vi "format_coords_str.vi"(2 "DEC str":string, 3 "RA str":string) -> (0 "%s DEC":string, 1 "%s RA":string)   [LabVIEW 2010]
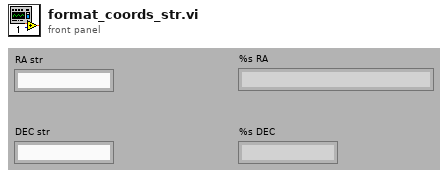
[diagram p1: front panel]
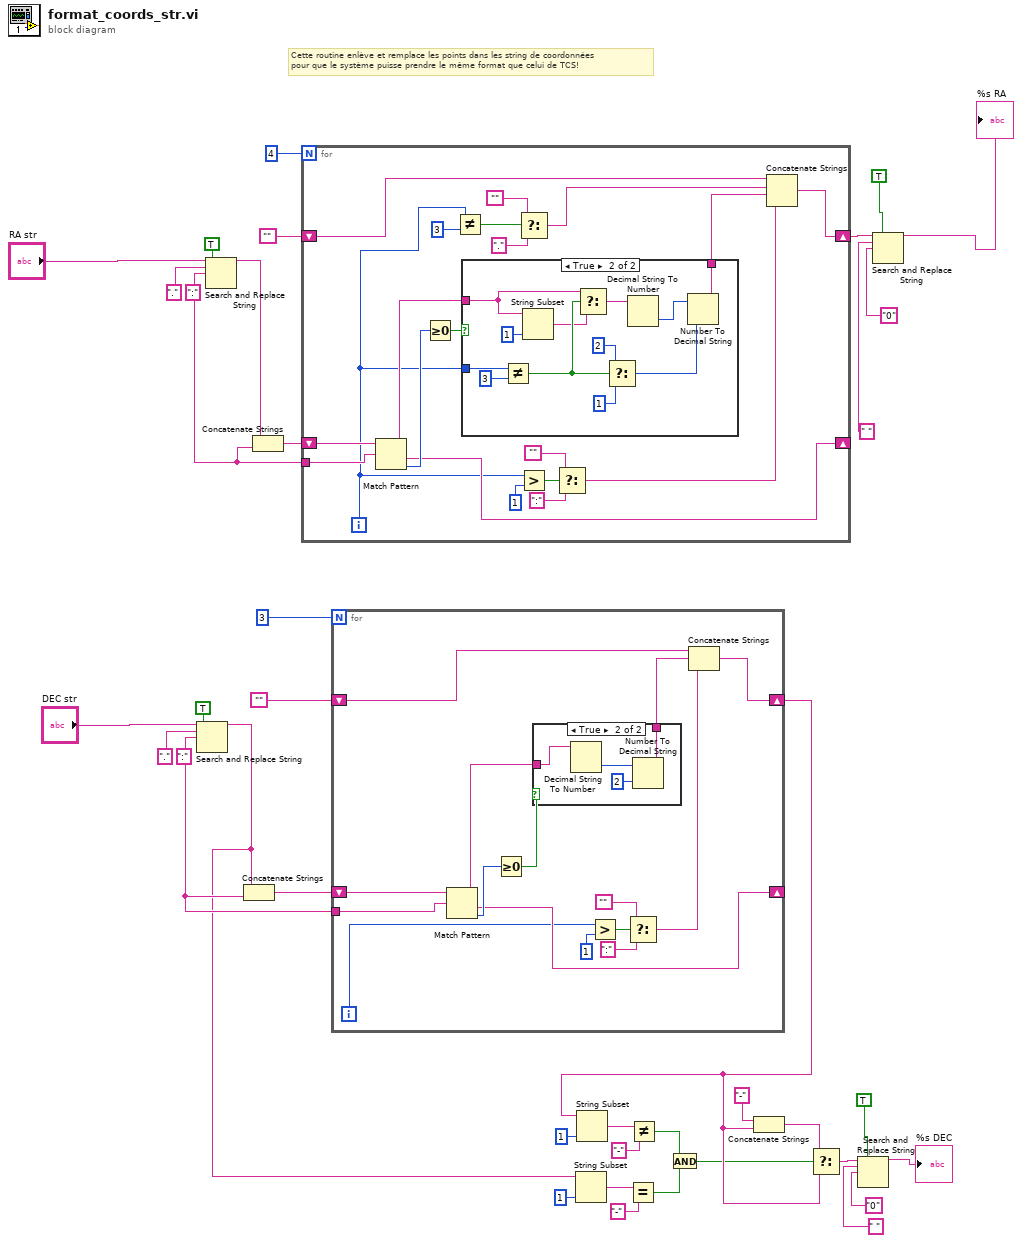
[diagram p0: block diagram]
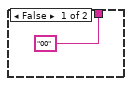
[diagram p2: hidden frame]
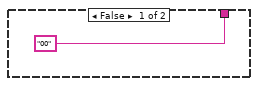
[diagram p3: hidden frame]
diagram:
  w15 = ":" ("replace string (\"\")")
  w31 = ":" ("replace string (\"\")")
  # "Cette routine enlève et remplace les points dans les string de coordonnées \npour que le système puisse prendre le même format que celui de TCS!"
  n1 = Search and Replace String(replace all?=TRUE ("replace all? (F)"), input string="DEC str", search string=".", replace string=w15) -> (result string=w1:string)  [unwired: 4 in, 3 out]
  n2 = Search and Replace String(replace all?=TRUE ("replace all? (F)"), input string="RA str", search string=".", replace string=w31) -> (result string=w33:string)  [unwired: 4 in, 3 out]
  n3 = Concatenate Strings(w1, w15) -> (w24:string)
  n4 = Concatenate Strings(w33, w31) -> (w34:string)
  n5 = for {
    N: 4 -> [_]
    shift-right: [w54] -> _
    shift-left: w34 -> [w57]
    shift-right: [w58] -> w32
    shift-left: "" -> [w41]
    tunnel: w31 -> [w51]
    i -> [w39]
    n6 = Match Pattern(string=w57, regular expression=w51) -> (before substring=w53:string, after substring=w54:string, offset past match=w55:i32)  [unwired: 1 in, 1 out]
    n7 = Greater Or Equal To 0?(x=w55) -> (x >= 0?=w56:bool)
    n8 = Not Equal?(x=w39, y=3) -> (x != y?=w43:bool)
    n9 = case shown="True" w56 {
      tunnel: w53 -> [_ w62]
      tunnel: ["00" w70] -> w52
      tunnel: w39 -> [_ w66]
      frame False {
      }
      frame True {
        n10 = Not Equal?(x=w66, y=3) -> (x != y?=w64:bool)
        n11 = String Subset(string=w62, length (rest)=1 ("length (rest)")) -> (substring=w61:string)  [unwired: 1 in]
        n12 = Select(t=w62, s=w64, f=w61) -> (s? t:f=w60:string)
        n13 = Select(t=i16 2 ("width (-)"), s=w64, f=i16 1 ("width (-)")) -> (s? t:f=w67:i16)
        n14 = Decimal String To Number(string=w60) -> (number=w71:i32)  [unwired: 2 in, 1 out]
        n15 = Number To Decimal String(number=w71, width (-)=w67) -> (decimal integer string=w70:string)
      }
    }
    n16 = Select(t="", s=w43, f="." ("replace string (\"\")")) -> (s? t:f=w40:string)
    n17 = Greater?(x=w39, y=1) -> (0:w49:bool)
    n18 = Select(t="", s=w49, f=":" ("replace string (\"\")")) -> (s? t:f=w46:string)
    n19 = Concatenate Strings(w41, w40, w52, w46) -> (w58:string)
  }
  n20 = for {
    N: 3 -> [_]
    shift-right: [w82] -> _
    shift-left: w24 -> [w85]
    shift-right: [w86] -> w3
    shift-left: "" -> [w80]
    tunnel: w15 -> [w78]
    i -> [w73]
    n21 = Match Pattern(string=w85, regular expression=w78) -> (before substring=w81:string, after substring=w82:string, offset past match=w83:i32)  [unwired: 1 in, 1 out]
    n22 = Greater Or Equal To 0?(x=w83) -> (x >= 0?=w84:bool)
    n23 = case shown="True" w84 {
      tunnel: w81 -> [_ w89]
      tunnel: ["00" w88] -> w79
      frame False {
      }
      frame True {
        n24 = Decimal String To Number(string=w89) -> (number=w90:i32)  [unwired: 2 in, 1 out]
        n25 = Number To Decimal String(number=w90, width (-)=i16 2) -> (decimal integer string=w88:string)
      }
    }
    n26 = Greater?(x=w73, y=1) -> (0:w76:bool)
    n27 = Select(t="", s=w76, f=":" ("replace string (\"\")")) -> (s? t:f=w72:string)
    n28 = Concatenate Strings(w80, w79, w72) -> (w86:string)
  }
  n29 = String Subset(string=w1, length (rest)=1 ("length (rest)")) -> (substring=w13:string)  [unwired: 1 in]
  n30 = String Subset(string=w3, length (rest)=1 ("length (rest)")) -> (substring=w10:string)  [unwired: 1 in]
  n31 = Equal?(x=w13, y="-") -> (x = y?=w7:bool)
  n32 = Not Equal?(x=w10, y="-") -> (x != y?=w8:bool)
  n33 = And(x=w8, y=w7) -> (x .and. y?=w2:bool)
  n34 = Concatenate Strings("-" ("string"), w3) -> (w4:string)
  n35 = Select(t=w4, s=w2, f=w3) -> (s? t:f=w5:string)
  n36 = Search and Replace String(replace all?=TRUE ("replace all? (F)"), input string=w5, search string=" ", replace string="0" ("replace string (\"\")")) -> (result string=→"%s DEC":string)  [unwired: 4 in, 3 out]
  n37 = Search and Replace String(replace all?=TRUE ("replace all? (F)"), input string=w32, search string=" ", replace string="0" ("replace string (\"\")")) -> (result string=→"%s RA":string)  [unwired: 4 in, 3 out]
